vi "String Split Cluster.vi"(0 "Array Str":string[](array[string]), 1 "Char":string) -> (5 "Array Cluster":cluster{"Table":string, "alias":string}[](array[cluster]))   [LabVIEW 2014]
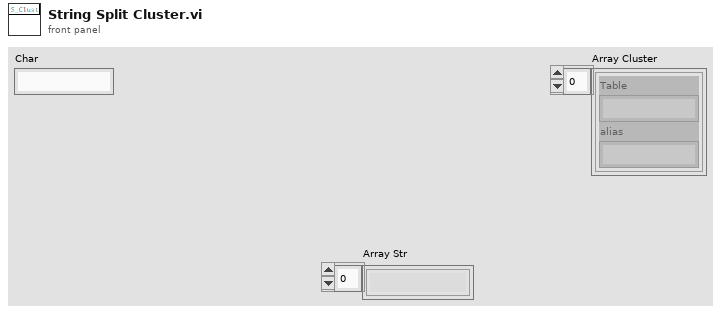
[diagram p1: front panel]
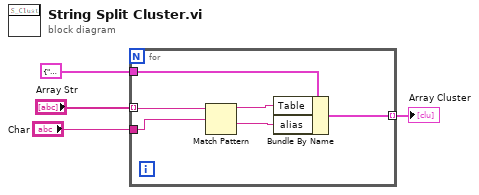
[diagram p0: block diagram]
diagram:
  n1 = for {
    tunnel: "Array Str" -> [w10] mode=indexing
    tunnel: "Char" -> [w9]
    tunnel: cluster{"Table":string, "alias":string} {"Table"="", "alias"=""} ("Tbale") -> [w8]
    tunnel: [w5] -> w1 mode=indexing
    n2 = Match Pattern(string=w10, regular expression=w9) -> (before substring=w7:string, after substring=w6:string)  [unwired: 1 in, 2 out]
    n3 = Bundle By Name(cluster=w8, "Table"=w7, "alias"=w6) -> (w5:cluster{"Table":string, "alias":string})
  }
  "Array Cluster" <- w1
